vi "Construct Protected Connection Reader.vi"(11 "Connection Reference":refnum<data-value>) -> (3 "ProtectedConnectionReader out":refnum<class "ProtectedConnectionReader.lvclass">)   [LabVIEW 2020, in "ProtectedConnectionReader.lvclass"]
uses:
  <vilib>/gpm_packages/@cs/Network-interface/Source/ProtectedConnectionReader/ProtectedConnectionReader.lvclass
  <vilib>/gpm_packages/@cs/Network-interface/Source/Connection Reference/Connection Reference/Connection Reference.lvclass
  <vilib>/gpm_packages/@cs/Network-interface/Source/ProtectedConnectionReader/ProtectedConnectionReader.lvclass/ProtectedConnectionReader.ctl
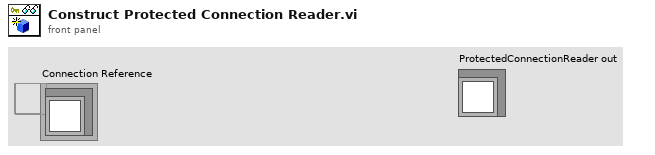
[diagram p1: front panel]
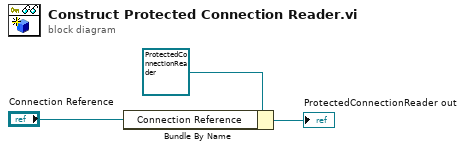
[diagram p0: block diagram]
diagram:
  n1 = Bundle By Name(cluster=refnum<class "ProtectedConnectionReader.lvclass"> refnum ("ProtectedConnectionReader in"), "Connection Reference"="Connection Reference") -> (→"ProtectedConnectionReader out":refnum<class "ProtectedConnectionReader.lvclass">)
